vi "Read Virt Instr CFG.vi"(8 "error in":errorcluster, 10 "Virt Instr CFG":path, 11 "File Provider in":refnum<class "File Provider.lvclass">) -> (0 "error out":errorcluster, 3 "File Provider out":refnum<class "File Provider.lvclass">)   [LabVIEW 2023, in "File Provider.lvlib" / "File Provider.lvclass"]
uses:
  File Provider.lvclass
  File Provider.lvclass/File Provider.ctl
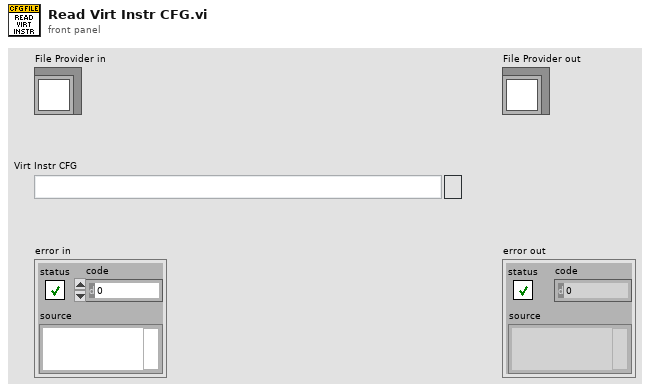
[diagram p1: front panel]
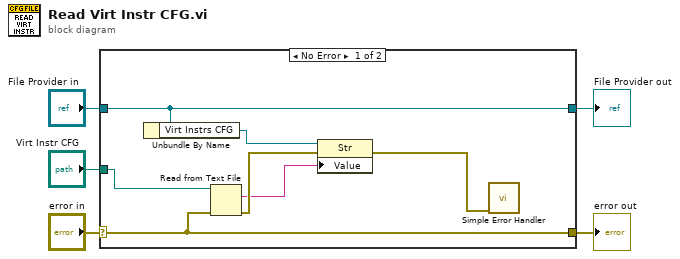
[diagram p0: block diagram]
diagram:
  n1 = case shown="No Error" "error in" {
    selector: "error in" -> [w12 w14]
    tunnel: [w12 w14] -> w4
    tunnel: [w10 w13] -> w2
    tunnel: "File Provider in" -> [w10 w13]
    tunnel: "Virt Instr CFG" -> [w11 _]
    frame No Error {
      n2 = Unbundle By Name(w10) -> ("Virt Instrs CFG"=w9:refnum<vi>)
      n3 = Read from Text File(file (use dialog)=w11, error in=w12) -> (text=w7:string, error out=w8:errorcluster)  [unwired: 2 in, 2 out]
      n4 = property class="Str"(reference=w9, error in=w8, "Value"=w7) -> (error out=w6:errorcluster)  [unwired: 1 out]
      n5 = call <vilib>:"Simple Error Handler.vi"("error in (no error)"=w6) -> ()  [unwired: 4 in, 5 out]
    }
    frame Error {
    }
  }
  "error out" <- w4
  "File Provider out" <- w2
